vi "UHR-Fleezers Control (host) - 16.2.2v2.vi"() -> ()   [LabVIEW 2014] (continued)
  n239 = call "IMAQ Create"("Image Name"="APD 1 Image", "Image Type"=w48) -> ("New Image"=w71:T2)  [unwired: 3 in, 1 out]
  n240 = call "IMAQ Create"("Image Name"="APD 2 Image", "Image Type"=w48) -> ("New Image"=w70:T2)  [unwired: 3 in, 1 out]
  n241 = call "IMAQ Create"("Image Name"="APD 3 Image", "Image Type"=w48) -> ("New Image"=w47:T2)  [unwired: 3 in, 1 out]
  n242 = call "IMAQ Create"("Image Name"="Det. X Image", "Image Type"=w48) -> ("New Image"=w69:T2)  [unwired: 3 in, 1 out]
  n243 = call "IMAQ Create"("Image Name"="Det. Y Image", "Image Type"=w48) -> ("New Image"=w68:T2)  [unwired: 3 in, 1 out]
  n244 = call-poly "VISA Configure Serial Port"("VISA resource name"=refnum<visa-resource-name> "COM1") -> ("VISA resource name out"=w15:refnum<visa-resource-name>, "error out"=w78:errorcluster)  [unwired: 5 in, 8 out]
  "Stage Control Serial Error" <- w78
  n245 = call-poly "VISA Configure Serial Port"("VISA resource name"=refnum<visa-resource-name> "COM6", "baud rate (9600)"=u32 115200, "stop bits (10: 1 bit)"=w65) -> ("VISA resource name out"=w63:refnum<visa-resource-name>, "error out"=w64:errorcluster)  [unwired: 4 in, 7 out]
  n246 = Bundle("New Image"=w71, "New Image"=w70, "New Image"=w47, "New Image"=w69, "New Image"=w68) -> (w67:T27)  [unwired: 1 in]
  n247 = node-c288() -> (w74:T28)  [unwired: 4 in]
  n248 = node-c288() -> (w87:T28)  [unwired: 4 out]
  n249 = node-c288() -> (w46:T28)  [unwired: 4 out]
  n250 = node-c288(3 ("Processor")) -> (w83:T28)  [unwired: 3 out]
  n251 = node-c288(2 ("Processor")) -> (w85:T28)  [unwired: 3 out]
  n252 = node-c288(i64 1 ("Period"), 1 ("Processor")) -> (w91:T28)  [unwired: 2 out]
  n253 = timed-loop "Run Scripts, including: stage motion" {
    tunnel: w78 -> [w430]
    tunnel: w15 -> [w431]
    tunnel: [w431] -> w77
    tunnel: [w430] -> w76
    timing: w74 -> [_]
    timing-out: [_] -> w73
    tunnel: w63 -> [w429]
    tunnel: w64 -> [w428]
    tunnel: w55 -> [w425]
    tunnel: w54 -> [w424]
    tunnel: w53 -> [w426]
    tunnel: w52 -> [w427]
    tunnel: w42 -> [w423]
    tunnel: w36 -> [w422]
    tunnel: w8 -> [w421]
    tunnel: w5 -> [w420]
    stop <- w432 stop-if-true
    n254 = node-c288() -> ()  [unwired: 1 in, 1 out]
    n255 = event shown="[32] \"Start slow f-ext\": Value Change" {
      selector: _ -> [_ _ _ _ _ _ _ _ _ _ _ _ _ _ _ _ _ _ _ _ _ _ _ _ _ _ _ _ _ _ _ _ _]
      dyn-events: _ -> [_ _ _ _ _ _ _ _ _ _ _ _ _ _ _ _ _ _ _ _ _ _ _ _ _ _ _ _ _ _ _ _ _]
      timeout: _ -> [_ _ _ _ _ _ _ _ _ _ _ _ _ _ _ _ _ _ _ _ _ _ _ _ _ _ _ _ _ _ _ _ _]
      tunnel: ["Set Position" "Move to Position" _ _ _ _ _ _ _ _ "Read Harvard" _ _ _ _ _ _ _ _ "Got ADig bead" "Force FB Data\nScript" _ _ _ "Got DNA bead" "Take Stepping Data" _ "Take Detection Laser\nImage" _ _ _ _ _] -> _
      tunnel: [_ _ _ _ _ _ _ _ _ _ _ _ _ _ _ _ _ _ _ _ _ _ _ _ _ _ _ _ _ w1446 _ _ _] -> w432
      tunnel: w430 -> [w451 w459 w472 w502 _ _ _ _ _ _ _ w646 w680 w706 w738 w832 w861 w993 w1020 _ w1056 _ _ _ _ _ _ _ _ _ _ _ _]
      tunnel: w431 -> [w452 w460 w473 w503 _ _ _ _ _ _ _ w647 w681 w707 w739 w833 w862 w994 w1021 _ w1057 _ _ _ _ _ _ _ _ _ _ _ _]
      tunnel: w429 -> [_ _ _ _ _ _ _ _ _ _ w631 _ _ _ _ _ _ _ _ _ _ _ _ _ _ _ _ _ _ _ _ _ _]
      tunnel: w428 -> [_ _ _ _ _ _ _ _ _ _ w630 _ _ _ _ _ _ _ _ _ _ _ _ _ _ _ _ _ _ _ _ _ _]
      tunnel: w427 -> [_ _ _ _ _ _ _ _ _ _ _ _ _ _ _ _ _ _ _ _ _ _ _ _ _ _ _ _ _ _ _ _ _]
      tunnel: w426 -> [_ _ _ _ _ _ _ _ _ _ _ _ _ _ _ _ _ _ _ _ _ _ _ _ _ _ _ _ _ _ _ _ _]
      tunnel: w425 -> [_ _ _ _ _ _ _ _ _ _ _ _ _ _ _ _ _ _ _ _ _ _ _ _ _ _ _ _ _ _ _ _ _]
      tunnel: w424 -> [_ _ _ _ _ _ _ _ _ _ _ _ _ _ _ _ _ _ _ _ _ _ _ _ _ _ _ _ _ _ _ _ _]
      tunnel: w423 -> [_ _ _ _ w530 w537 w565 w584 _ _ _ _ _ _ _ _ _ _ _ _ _ _ _ _ _ _ _ _ _ w1445 _ _ _]
      tunnel: w422 -> [_ _ _ _ _ _ _ _ _ _ _ _ _ _ _ _ _ _ _ _ _ w1104 w1117 _ _ _ _ _ w1312 _ _ _ _]
      tunnel: w421 -> [_ _ _ _ _ _ _ _ _ _ _ _ _ _ _ _ _ _ _ _ _ _ _ _ _ _ _ _ _ _ w1456 _ _]
      tunnel: w420 -> [_ _ _ _ _ _ _ _ _ _ _ _ _ _ _ _ _ _ _ _ _ _ _ _ _ _ _ _ _ _ w1451 _ _]
      event "Set Position", "Set Position 2", "Set Position 3", "Set Position 4", "Set Position 5", "Set Position 1", "Set Position 6": Value Change {
        n256 = event-data() -> ()  [unwired: 1 in, 5 out]
        n257 = Build Array("Set Position 1", "Set Position 2", "Set Position 3", "Set Position 4", "Set Position 5", "Set Position 6") -> (w450:bool[])
        n258 = Boolean Array To Number(Boolean array=w450) -> (number=w449:u32)
        n259 = Logarithm Base 2(1:w449) -> (0:w441:dbl)
        n260 = call "Read Stage Position.vi"("error in"=w451, "VISA resource name in"=w452) -> ("Current Position"=w456:cluster{dbl, dbl, dbl}, "error out"=w455:errorcluster)  [unwired: 2 out]
        n261 = Decrement(x="Position") -> (x-1=w439:dbl)
        n262 = Greater Or Equal?(x=w441, y=0.0) -> (x >= y?=w442:bool)
        n263 = Cluster To Array(cluster=w456) -> (array=w453:dbl[])
        n264 = local write "Stage Control Serial Error"(w455) -> ()
        n265 = Select(t=w441, s=w442, f=w439) -> (s? t:f=w438:dbl)
        n266 = Increment(x=w438) -> (x+1=w437:dbl)
        n267 = Build Array (concatenate)(w437, w453) -> (w436:dbl[])
        n268 = Replace Array Subset(array="Saved Stage Positions", new element=w436, index (row)=w438) -> (w454:dbl[][])  [unwired: 1 in]
        n269 = local write "Saved Stage Positions"(w454) -> ()
      }
      event "Move to Position": Value Change {
        n270 = event-data() -> ()  [unwired: 1 in, 5 out]
        n271 = flat-sequence {
          tunnel: w460 -> [w464]
          tunnel: w459 -> [w463]
          frame #0 {
            n272 = local read "Saved Stage Positions"() -> (w466:dbl[][])
            n273 = local read "Position"() -> (w465:dbl)
            n274 = local write "Stage Moving"(TRUE ("Stage Moving")) -> ()
            n275 = call "move to saved stage position.vi"("error in"=w463, "Stage VISA resource name in"=w464, "Position"=w465, "Saved Stage Positions"=w466) -> ("error out"=w462:errorcluster)  [unwired: 1 out]
            n276 = local write "Stage Control Serial Error"(w462) -> ()
          }
          frame #1 {
            n277 = call <vilib>:"Beep.vi"() -> ()  [unwired: 3 in, 9 out]
            n278 = local write "Stage Moving"(FALSE ("Stage Moving")) -> ()
          }
        }
      }
      event "Move Cap. 1 (DNA Bottom)": Value Change {
        n279 = event-data() -> ()  [unwired: 1 in, 5 out]
        n280 = local write "Move Cap. 1 (DNA Bottom)"(FALSE ("Move Cap. 1 (DNA Right)")) -> ()
        n281 = flat-sequence {
          tunnel: w472 -> [w475]
          tunnel: w473 -> [w476]
          tunnel: [w476] -> w470
          tunnel: [w475] -> w469
          tunnel: w470 -> [w478]
          tunnel: w469 -> [w477]
          frame #0 {
            n282 = property on="Sample Channel\nFlow" class="Bool (strict)"("Val(Sgnl)"="Cap 1 Samp Flow ON") -> ()  [unwired: 2 in, 2 out]
          }
          frame #1 {
            n283 = local read "Saved Stage Positions"() -> (w488:dbl[][])
            n284 = local write "Stage Moving"(TRUE ("Stage Moving")) -> ()
            n285 = Array Subset(array=w488, index (row)=0 ("index"), length (row)=1 ("length"), index (col)=1 ("index"), length (col)=3 ("length")) -> (w485:dbl[][])
            n286 = Reshape Array(w485, 3 ("dimension size")) -> (w483:dbl[])
            n287 = Array To Cluster(array=w483) -> (cluster=w482:cluster{"[0]":dbl, "[1]":dbl, "[2]":dbl})
            n288 = call "Set Stage Position.vi"("Position"=w482, "error in"=w477, "VISA resource name in"=w478) -> ("error out"=w481:errorcluster)  [unwired: 2 out]
            n289 = local write "Stage Control Serial Error"(w481) -> ()
          }
          frame #2 {
            n290 = local write "Stage Moving"(FALSE ("Stage Moving")) -> ()
            n291 = case shown="True" "Cap 1 Flow ON" {
              frame False {
              }
              frame True {
                n292 = property on="Inject Pump 1" class="Bool (strict)"("Val(Sgnl)"=TRUE ("Value (Signaling)")) -> ()  [unwired: 2 in, 2 out]
              }
            }
            n293 = call <vilib>:"Beep.vi"() -> ()  [unwired: 3 in, 9 out]
          }
          frame #3 {
            n294 = property on="Sample Channel\nFlow" class="Bool (strict)"("Val(Sgnl)"=FALSE ("Value (Signaling)")) -> ()  [unwired: 2 in, 2 out]
            n295 = local read "Cap. 2 BD T1?\n(ADig T1, DNA T2)"() -> (w495:bool)
            n296 = case shown="True" w495 {
              tunnel: "Cap 1 T ON" -> [w497 w498]
              frame False {
                n297 = property on="Trap 1 (ON/OFF)" class="Bool (strict)"("Val(Sgnl)"=w497) -> ()  [unwired: 2 in, 2 out]
              }
              frame True {
                n298 = property on="Trap 2 (ON/OFF)" class="Bool (strict)"("Val(Sgnl)"=w498) -> ()  [unwired: 2 in, 2 out]
              }
            }
            n299 = property on="Got DNA bead" class="Bool"("Key Focus"=TRUE) -> ()  [unwired: 2 in, 2 out]
          }
        }
      }
      event "Move Cap. 2 (ADig Top)": Value Change {
        n300 = event-data() -> ()  [unwired: 1 in, 5 out]
        n301 = local write "Move Cap. 2 (ADig Top)"(FALSE ("Move Cap. 2 (ADig Left)")) -> ()
        n302 = flat-sequence {
          tunnel: w502 -> [w505]
          tunnel: w503 -> [w506]
          tunnel: [w506] -> w500
          tunnel: [w505] -> w499
          tunnel: w500 -> [w509]
          tunnel: w499 -> [w508]
          frame #0 {
            n303 = property on="Sample Channel\nFlow" class="Bool (strict)"("Val(Sgnl)"="Cap 2 Samp Flow ON") -> ()  [unwired: 2 in, 2 out]
          }
          frame #1 {
            w507 = FALSE ("Value (Signaling)")
            n304 = local read "Saved Stage Positions"() -> (w519:dbl[][])
            n305 = local write "Stage Moving"(TRUE ("Stage Moving")) -> ()
            n306 = Array Subset(array=w519, index (row)=1 ("index"), length (row)=1 ("length"), index (col)=1 ("index"), length (col)=3 ("length")) -> (w516:dbl[][])
            n307 = Reshape Array(w516, 3 ("dimension size")) -> (w514:dbl[])
            n308 = property on="Trap 1 (ON/OFF)" class="Bool (strict)"("Val(Sgnl)"=w507) -> ()  [unwired: 2 in, 2 out]
            n309 = property on="Trap 1 (ON/OFF)" class="Bool (strict)"("Val(Sgnl)"=w507) -> ()  [unwired: 2 in, 2 out]
            n310 = Array To Cluster(array=w514) -> (cluster=w513:cluster{"[0]":dbl, "[1]":dbl, "[2]":dbl})
            n311 = call "Set Stage Position.vi"("Position"=w513, "error in"=w508, "VISA resource name in"=w509) -> ("error out"=w512:errorcluster)  [unwired: 2 out]
            n312 = local write "Stage Control Serial Error"(w512) -> ()
          }
          frame #2 {
            n313 = local write "Stage Moving"(FALSE ("Stage Moving")) -> ()
            n314 = call <vilib>:"Beep.vi"() -> ()  [unwired: 3 in, 9 out]
            n315 = case shown="True" "Cap 2 Flow ON" {
              frame False {
              }
              frame True {
                n316 = property on="Inject Pump 3" class="Bool (strict)"("Val(Sgnl)"=TRUE ("Value (Signaling)")) -> ()  [unwired: 2 in, 2 out]
              }
            }
          }
          frame #3 {
            n317 = property on="Sample Channel\nFlow" class="Bool (strict)"("Val(Sgnl)"=FALSE ("Value (Signaling)")) -> ()  [unwired: 2 in, 2 out]
            n318 = case shown="False" "Cap. 2 BD T1?\n(ADig T1, DNA T2)" {
              tunnel: "Cap 2 T ON" -> [w528 w529]
              frame False {
                n319 = property on="Trap 2 (ON/OFF)" class="Bool (strict)"("Val(Sgnl)"=w528) -> ()  [unwired: 2 in, 2 out]
              }
              frame True {
                n320 = property on="Trap 1 (ON/OFF)" class="Bool (strict)"("Val(Sgnl)"=w529) -> ()  [unwired: 2 in, 2 out]
              }
            }
            n321 = property on="Got ADig bead" class="Bool"("Key Focus"=TRUE) -> ()  [unwired: 2 in, 2 out]
          }
        }
      }
      event "Send string\nto Blue Laser": Value Change {
        n322 = event-data() -> ()  [unwired: 1 in, 5 out]
        n323 = flat-sequence {
          tunnel: w530 -> [w531]
          frame #0 {
            n324 = call "serial write macro.vi"("String"="command string", "Delay (ms)"="Delay (ms)", "VISA resource name"=w531) -> ("read buffer"=→"read blue buffer":string, "error out"=→"Blue Error Out":errorcluster)  [unwired: 1 out]
            "command string sent" <- "command string"
          }
          frame #1 {
            n325 = local write "Send string\nto Blue Laser"(FALSE ("Send string")) -> ()
          }
        }
      }
      event "Get Blue Laser State": Value Change {
        n326 = event-data() -> ()  [unwired: 1 in, 5 out]
        n327 = local read "Delay (ms)"() -> (w538:i32)
        n328 = flat-sequence {
          tunnel: w538 -> [w546]
          tunnel: w537 -> [w549]
          tunnel: [w547] -> w542
          tunnel: [w546] -> w541
          tunnel: [w556] -> w540
          tunnel: [w553] -> w539
          tunnel: w542 -> [w554]
          tunnel: w541 -> [w553]
          tunnel: w540 -> [w562]
          tunnel: w539 -> [w560]
          frame #0 {
            w544 = "l?"
            n329 = local write "command string sent"(w544) -> ()
            n330 = call "serial write macro.vi"("String"=w544, "Delay (ms)"=w546, "VISA resource name"=w549) -> ("read buffer"=w545:string, "VISA resource name out"=w547:refnum<visa-resource-name>)  [unwired: 1 out]
            n331 = Decimal String To Number(string=w545) -> (number=w548:i32)  [unwired: 2 in, 1 out]
            n332 = Not Equal To 0?(x=w548) -> (x != 0?=→"Laser On":bool)
            n333 = local write "read blue buffer"(w545) -> ()
          }
          frame #1 {
            w551 = "games?" ("String")
            n334 = local write "command string sent"(w551) -> ()
            n335 = call "serial write macro.vi"("String"=w551, "Delay (ms)"=w553, "VISA resource name"=w554) -> ("read buffer"=w552:string, "VISA resource name out"=w556:refnum<visa-resource-name>)  [unwired: 1 out]
            n336 = Decimal String To Number(string=w552) -> (number=w555:i32)  [unwired: 2 in, 1 out]
            n337 = local write "read blue buffer"(w552) -> ()
            n338 = Not Equal To 0?(x=w555) -> (x != 0?=→"Analog Modulation":bool)
          }
          frame #2 {
            w558 = "gdmes?" ("String")
            n339 = local write "command string sent"(w558) -> ()
            n340 = call "serial write macro.vi"("String"=w558, "Delay (ms)"=w560, "VISA resource name"=w562) -> ("read buffer"=w559:string)  [unwired: 2 out]
            n341 = Decimal String To Number(string=w559) -> (number=w561:i32)  [unwired: 2 in, 1 out]
            n342 = Not Equal To 0?(x=w561) -> (x != 0?=→"Digital Modulation":bool)
            n343 = local write "read blue buffer"(w559) -> ()
          }
          frame #3 {
            n344 = local write "Get Blue Laser State"(FALSE) -> ()
          }
        }
      }
      event "Blue Laser Power (mW)\n(Constant Power Mode)", "Blue Laser Modulation\nPower (mW)": Value Change {
        n345 = event-data() -> ()  [unwired: 1 in, 5 out]
        n346 = flat-sequence {
          tunnel: w565 -> [w571]
          tunnel: [w569] -> w564
          tunnel: w564 -> [w578]
          frame #0 {
            n347 = local read "Delay (ms)"() -> (w570:i32)
            n348 = Concatenate Strings("slmp " ("string"), "Blue Laser Modulation\nPower (mW)") -> (w566:string)
            n349 = call "serial write macro.vi"("String"=w566, "Delay (ms)"=w570, "VISA resource name"=w571) -> ("read buffer"=w567:string, "error out"=w568:errorcluster, "VISA resource name out"=w569:refnum<visa-resource-name>)
            n350 = local write "command string sent"(w566) -> ()
            n351 = local write "read blue buffer"(w567) -> ()
            n352 = local write "Blue Error Out"(w568) -> ()
          }
          frame #1 {
            n353 = local read "Delay (ms)"() -> (w577:i32)
            n354 = Concatenate Strings("p " ("string"), "Blue Laser Power (mW)\n(Constant Power Mode)") -> (w574:string)
            n355 = call "serial write macro.vi"("String"=w574, "Delay (ms)"=w577, "VISA resource name"=w578) -> ("read buffer"=w575:string, "error out"=w576:errorcluster)  [unwired: 1 out]
            n356 = local write "command string sent"(w574) -> ()
            n357 = local write "read blue buffer"(w575) -> ()
            n358 = local write "Blue Error Out"(w576) -> ()
          }
        }
      }
      event "Laser interlacing mode", "Blue Laser Modulation Mode", "Blue Laser ON": Value Change {
        n359 = event-data() -> ()  [unwired: 1 in, 5 out]
        n360 = flat-sequence {
          tunnel: w584 -> [w589]
          tunnel: [w588] -> w581
          tunnel: [w594] -> w583
          tunnel: w581 -> [w597]
          tunnel: w583 -> [w609]
          tunnel: [w603] -> w582
          tunnel: w582 -> [w616]
          frame #0 {
            n361 = local read "Blue Laser ON"() -> (w586:bool)
            n362 = local read "Delay (ms)"() -> (w587:i32)
            n363 = case shown="False" w586 {
              tunnel: ["l0" "l1"] -> w585
              frame False {
              }
              frame True {
              }
            }
            n364 = call "serial write macro.vi"("String"=w585, "Delay (ms)"=w587, "VISA resource name"=w589) -> ("error out"=w590:errorcluster, "VISA resource name out"=w588:refnum<visa-resource-name>)  [unwired: 1 out]
            n365 = local write "Blue Error Out"(w590) -> ()
          }
          frame #1 {
            n366 = local read "Laser interlacing mode"() -> (w599:enum32{"Laser ON", "Laser OFF", "Interlace"})
            n367 = case shown="\"Laser ON\"" w599 {
              tunnel: ["cp" "em" "l0"] -> w593
              frame "Laser ON" {
              }
              frame "Interlace" {
              }
              frame "Laser OFF", Default {
              }
            }
            n368 = local read "Delay (ms)"() -> (w598:i32)
            n369 = call "serial write macro.vi"("String"=w593, "Delay (ms)"=w598, "VISA resource name"=w597) -> ("read buffer"=w595:string, "error out"=w596:errorcluster, "VISA resource name out"=w594:refnum<visa-resource-name>)
            n370 = local write "command string sent"(w593) -> ()
            n371 = local write "read blue buffer"(w595) -> ()
            n372 = local write "Blue Error Out"(w596) -> ()
          }
          frame #2 {
            n373 = case shown="\"Analog Modulation\"" "Blue Laser Modulation Mode" {
              tunnel: ["sdmes 0" "sdmes 1" "sdmes 1"] -> w604
              frame "Analog Modulation" {
              }
              frame "Digital + Analog Modulation" {
              }
              frame "Digital Modulation", Default {
              }
            }
            n374 = local read "Delay (ms)"() -> (w607:i32)
            n375 = call "serial write macro.vi"("String"=w604, "Delay (ms)"=w607, "VISA resource name"=w609) -> ("read buffer"=w605:string, "error out"=w606:errorcluster, "VISA resource name out"=w603:refnum<visa-resource-name>)
            n376 = local write "command string sent"(w604) -> ()
            n377 = local write "read blue buffer"(w605) -> ()
            n378 = local write "Blue Error Out"(w606) -> ()
          }
          frame #3 {
            n379 = local read "Blue Laser Modulation Mode"() -> (w618:string)
            n380 = case shown="\"Digital Modulation\", Default" w618 {
              tunnel: ["sames 1" "sames 1" "sames 0"] -> w614
              frame "Analog Modulation" {
              }
              frame "Digital + Analog Modulation" {
              }
              frame "Digital Modulation", Default {
              }
            }
            n381 = local read "Delay (ms)"() -> (w617:i32)
            n382 = local write "command string sent"(w614) -> ()
            n383 = call "serial write macro.vi"("String"=w614, "Delay (ms)"=w617, "VISA resource name"=w616) -> ("read buffer"=w615:string, "error out"=w613:errorcluster)  [unwired: 1 out]
            n384 = local write "read blue buffer"(w615) -> ()
            n385 = local write "Blue Error Out"(w613) -> ()
          }
        }
      }
      event "All excitation lasers OFF": Value Change {
        n386 = event-data() -> ()  [unwired: 1 in, 5 out]
        n387 = flat-sequence {
          frame #0 {
            w623 = FALSE ("Red Laser ON")
            n388 = local write "All excitation lasers OFF"(FALSE ("All excitation lasers OFF")) -> ()
            n389 = local write "Blue Laser ON"(w623) -> ()
            n390 = local write "Red Laser ON"(w623) -> ()
          }
          frame #1 {
            n391 = property on="Green Laser ON" class="Bool (strict)"("Val(Sgnl)"=FALSE ("Value (Signaling)")) -> ()  [unwired: 2 in, 2 out]
          }
        }
      }
      event "Start ALEX": Value Change {
        n392 = event-data() -> ()  [unwired: 1 in, 5 out]
        n393 = flat-sequence {
          frame #0 {
            n394 = property on="ALEX ON" class="Bool (strict)"("Val(Sgnl)"=FALSE ("Value (Signaling)")) -> ()  [unwired: 2 in, 2 out]
          }
          frame #1 {
            w626 = TRUE ("Value (Signaling)")
            n395 = local write "Red Laser ON"(w626) -> ()
            n396 = local write "Start ALEX"(FALSE ("Start ALEX")) -> ()
            n397 = property on="ALEX ON" class="Bool (strict)"("Val(Sgnl)"=w626) -> ()  [unwired: 2 in, 2 out]
          }
          frame #2 {
            n398 = property on="Green Laser ON" class="Bool (strict)"("Val(Sgnl)"=TRUE ("Value (Signaling)")) -> ()  [unwired: 2 in, 2 out]
          }
        }
      }
      event "Read Harvard": Value Change {
        n399 = event-data() -> ()  [unwired: 1 in, 5 out]
        n400 = Concatenate Strings("write buffer", "\r") -> (w633:string)
        n401 = VISA Write(VISA resource name=w631, write buffer=w633, error in (no error)=w630) -> (VISA resource name out=w642:refnum<visa-resource-name>, error out=w641:errorcluster)  [unwired: 1 out]
        n402 = stacked-sequence {
          tunnel: [w645] -> w640
          tunnel: w642 -> [w645]
          tunnel: w641 -> [w644]
          tunnel: [w644] -> w635
          frame #0 {
            n403 = Wait (ms)(milliseconds to wait=50) -> ()  [unwired: 1 out]
          }
        }
        n404 = property class="Instr"(reference=w640, error in=w635) -> (reference out=w639:refnum<visa-resource-name>, error out=w637:errorcluster, "Serial Settings:Number of Bytes at Serial Port"=w638:u32)
        "Serial Settings:Number of Bytes at Serial Port" <- w638
        n405 = VISA Read(VISA resource name=w639, byte count=w638, error in (no error)=w637) -> (read buffer=w636:string)  [unwired: 3 out]
        "read buffer" <- w636
        n406 = Fract/Exp String To Number(string=w636) -> ()  [unwired: 5 out]
      }
      event "+z", "-z": Value Change {
        n407 = event-data() -> ()  [unwired: 1 in, 5 out]
        n408 = flat-sequence {
          tunnel: w646 -> [w668]
          tunnel: w647 -> [w648]
          frame #0 {
            n409 = call "Read Stage Position.vi"("error in"=w668, "VISA resource name in"=w648) -> ("Current Position"=w653:cluster{dbl, dbl, dbl}, "error out"=w666:errorcluster, "VISA resource name out"=w667:refnum<visa-resource-name>)  [unwired: 1 out]
            n410 = local read "Saved Stage Positions"() -> (w677:dbl[][])
            n411 = Divide(x="z nudge increment (um)", y=1000.0) -> (x/y=w665:dbl)
            n412 = Boolean To (0,1)(Boolean="+z") -> (0, 1=w657:i16)
            n413 = Boolean To (0,1)(Boolean="-z") -> (0, 1=w658:i16)
            n414 = Array Subset(array=w677, index (row)=1 ("index"), length (row)=1 ("length"), index (col)=1 ("index"), length (col)=3 ("length")) -> (w674:dbl[][])
            n415 = Multiply(x=w657, y=w665) -> (x*y=w661:dbl)
            n416 = Multiply(x=w658, y=w665) -> (x*y=w659:dbl)
            n417 = Unbundle(w653) -> (w651:dbl, w650:dbl, w654:dbl)
            n418 = Negate(x=w659) -> (-x=w660:dbl)
            n419 = Reshape Array(w674, 3 ("dimension size")) -> (w672:dbl[])
            n420 = Add(x=w661, y=w660) -> (x+y=w662:dbl)
            n421 = Array To Cluster(array=w672) -> ()  [unwired: 1 out]
            n422 = Add(x=w662, y=w654) -> (x+y=w652:dbl)
            n423 = Bundle(cluster=w653, w651, w650, w652) -> (w649:cluster{dbl, dbl, dbl})
            n424 = call "Set Stage Position.vi"("Position"=w649, "error in"=w666, "VISA resource name in"=w667) -> ("error out"=w671:errorcluster)  [unwired: 2 out]
            n425 = local write "Stage Moving"(TRUE ("Stage Moving")) -> ()
            n426 = local write "Stage Control Serial Error"(w671) -> ()
          }
          frame #1 {
            n427 = local write "Stage Moving"(FALSE ("Stage Moving")) -> ()
          }
        }
      }
      event "-y", "+y": Value Change {
        n428 = event-data() -> ()  [unwired: 1 in, 5 out]
        n429 = flat-sequence {
          tunnel: w680 -> [w704]
          tunnel: w681 -> [w687]
          frame #0 {
            n430 = call "Read Stage Position.vi"("error in"=w704, "VISA resource name in"=w687) -> ("Current Position"=w690:cluster{dbl, dbl, dbl}, "error out"=w702:errorcluster, "VISA resource name out"=w703:refnum<visa-resource-name>)  [unwired: 1 out]
            n431 = Divide(x="y nudge increment (um", y=1000.0) -> (x/y=w701:dbl)
            n432 = Boolean To (0,1)(Boolean="+y") -> (0, 1=w693:i16)
            n433 = Boolean To (0,1)(Boolean="-y") -> (0, 1=w694:i16)
            n434 = Multiply(x=w693, y=w701) -> (x*y=w697:dbl)
            n435 = Multiply(x=w694, y=w701) -> (x*y=w695:dbl)
            n436 = Unbundle(w690) -> (w689:dbl, w684:dbl, w686:dbl)
            n437 = Negate(x=w695) -> (-x=w696:dbl)
            n438 = Add(x=w697, y=w696) -> (x+y=w698:dbl)
            n439 = Add(x=w698, y=w684) -> (x+y=w685:dbl)
            n440 = Bundle(cluster=w690, w689, w685, w686) -> (w688:cluster{dbl, dbl, dbl})
            n441 = call "Set Stage Position.vi"("Position"=w688, "error in"=w702, "VISA resource name in"=w703) -> ("error out"=w683:errorcluster)  [unwired: 2 out]
            n442 = local write "Stage Control Serial Error"(w683) -> ()
            n443 = local write "Stage Moving"(TRUE ("Stage Moving")) -> ()
          }
          frame #1 {
            n444 = local write "Stage Moving"(FALSE ("Stage Moving")) -> ()
          }
        }
      }
      event "-x", "+x": Value Change {
        n445 = event-data() -> ()  [unwired: 1 in, 5 out]
        n446 = flat-sequence {
          tunnel: w706 -> [w730]
          tunnel: w707 -> [w714]
          frame #0 {
            n447 = call "Read Stage Position.vi"("error in"=w730, "VISA resource name in"=w714) -> ("Current Position"=w716:cluster{dbl, dbl, dbl}, "error out"=w728:errorcluster, "VISA resource name out"=w729:refnum<visa-resource-name>)  [unwired: 1 out]
            n448 = Divide(x="x nudge increment (um)", y=1000.0) -> (x/y=w727:dbl)
            n449 = Boolean To (0,1)(Boolean="+x") -> (0, 1=w719:i16)
            n450 = Boolean To (0,1)(Boolean="-x") -> (0, 1=w720:i16)
            n451 = Multiply(x=w719, y=w727) -> (x*y=w723:dbl)
            n452 = Multiply(x=w720, y=w727) -> (x*y=w721:dbl)
            n453 = Unbundle(w716) -> (w708:dbl, w710:dbl, w713:dbl)
            n454 = Negate(x=w721) -> (-x=w722:dbl)
            n455 = Add(x=w723, y=w722) -> (x+y=w724:dbl)
            n456 = Add(x=w724, y=w708) -> (x+y=w709:dbl)
            n457 = Bundle(cluster=w716, w709, w710, w713) -> (w715:cluster{dbl, dbl, dbl})
            n458 = call "Set Stage Position.vi"("Position"=w715, "error in"=w728, "VISA resource name in"=w729) -> ("error out"=w711:errorcluster)  [unwired: 2 out]
            n459 = local write "Stage Control Serial Error"(w711) -> ()
            n460 = local write "Stage Moving"(TRUE ("Stage Moving")) -> ()
          }
          frame #1 {
            n461 = local write "Stage Moving"(FALSE ("Stage Moving")) -> ()
          }
        }
      }
      event "Cal/Data Acq. Spot": Value Change {
        n462 = event-data() -> ()  [unwired: 1 in, 5 out]
        n463 = flat-sequence {
          tunnel: w738 -> [w742]
          tunnel: w739 -> [w743]
          tunnel: [w743] -> w735
          tunnel: [w742] -> w734
          tunnel: w735 -> [w748]
          tunnel: w734 -> [w747]
          tunnel: ["Cal @ (MHz)"] -> w732
          tunnel: [w752] -> w736
          tunnel: w732 -> [w752]
          tunnel: w736 -> [w764]
          tunnel: ["W/ Offset 1"] -> w733
          tunnel: w736 -> [w785]
          tunnel: w733 -> [w783]
          frame #0 {
            n464 = property on="Sample Channel\nFlow" class="Bool (strict)"("Val(Sgnl)"="Daq spot flow on") -> ()  [unwired: 2 in, 2 out]
            n465 = Wait (ms)(milliseconds to wait=u32 250) -> ()  [unwired: 1 out]
          }
          frame #1 {
            n466 = local read "Saved Stage Positions"() -> (w745:dbl[][])
            n467 = property on="Trap Delta (MHz)" class="DigNum (strict)"("Val(Sgnl)"="Cal @ (MHz)") -> ()  [unwired: 2 in, 2 out]
            n468 = local write "Stage Moving"(TRUE ("Stage Moving")) -> ()
            n469 = call "move to saved stage position.vi"("error in"=w747, "Stage VISA resource name in"=w748, "Position"="Cal Stage Position", "Saved Stage Positions"=w745) -> ("error out"=w746:errorcluster)  [unwired: 1 out]
            n470 = local write "Stage Control Serial Error"(w746) -> ()
          }
          frame #2 {
            n471 = local write "Stage Moving"(FALSE ("Stage Moving")) -> ()
            n472 = property on="Sample Channel\nFlow" class="Bool (strict)"("Val(Sgnl)"="Flow ON during cal?") -> ()  [unwired: 2 in, 2 out]
            n473 = call <vilib>:"Beep.vi"() -> ()  [unwired: 3 in, 9 out]
          }
          frame #3 {
            n474 = Wait (ms)(milliseconds to wait=u32 1000) -> ()  [unwired: 1 out]
          }
          frame #4 {
            n475 = case shown="True" "Active cal after cal?" {
              frame False {
              }
              frame True {
                n476 = local write "Active Cal"(TRUE ("Active Cal")) -> ()
                n477 = Wait (ms)(milliseconds to wait=u32 8000) -> ()  [unwired: 1 out]
              }
            }
          }
          frame #5 {
            n478 = property on="Save Calibration" class="Bool (strict)"("Val(Sgnl)"=TRUE ("Value (Signaling)")) -> ()  [unwired: 2 in, 2 out]
          }
          frame #6 {
            n479 = Wait (ms)(milliseconds to wait=u32 2000) -> ()  [unwired: 1 out]
          }
          frame #7 {
            # "Check to see if \nsaving done"
            n480 = while {
              stop <- w760 stop-if-true
              n481 = local read "Saving..."() -> (w761:bool)
              n482 = Wait (ms)(milliseconds to wait=u32 100) -> ()  [unwired: 1 out]
              n483 = Not(x=w761) -> (.not. x?=w760:bool)
            }
          }
          frame #8 {
            n484 = case shown="True" "W/ Offset 1" {
              tunnel: w764 -> [_ w765]
              frame False {
              }
              frame True {
                n485 = stacked-sequence {
                  tunnel: w765 -> [_ _ _ _ _ _ _ w782]
                  frame #0 {
                    n486 = property on="Trap Delta (MHz)" class="DigNum (strict)"("Val(Sgnl)"="Offset 1 Start (MHz)") -> ()  [unwired: 2 in, 2 out]
                    n487 = Replace Array Subset(array=u32[] [0] ("Index Values"), new element="Offset 1 Set", index=0) -> (w766:u32[])
                    n488 = property on="Saved AOD Raster Scan Parameter Sets" class="Arr (strict)"("Index Values"=w766) -> ()  [unwired: 2 in, 2 out]
                  }
                  frame #1 {
                    n489 = Wait (ms)(milliseconds to wait=u32 200) -> ()  [unwired: 1 out]
                  }
                  frame #2 {
                    n490 = property on="Load parameters" class="Bool (strict)"("Val(Sgnl)"=TRUE ("Value (Signaling)")) -> ()  [unwired: 2 in, 2 out]
                  }
                  frame #3 {
                    n491 = Wait (ms)(milliseconds to wait=u32 200) -> ()  [unwired: 1 out]
                  }
                  frame #4 {
                    n492 = property on="Trap Raster Scan" class="Bool (strict)"("Val(Sgnl)"=TRUE ("Value (Signaling)")) -> ()  [unwired: 2 in, 2 out]
                  }
                  frame #5 {
                    n493 = Wait (ms)(milliseconds to wait=u32 2000) -> ()  [unwired: 1 out]
                  }
                  frame #6 {
                    n494 = while {
                      stop <- w779 stop-if-true
                      n495 = local read "Raster Scanning..."() -> (w781:bool)
                      n496 = local read "Saving..."() -> (w777:bool)
                      n497 = Wait (ms)(milliseconds to wait=u32 100) -> ()  [unwired: 1 out]
                      n498 = Not(x=w777) -> (.not. x?=w776:bool)
                      n499 = Not(x=w781) -> (.not. x?=w778:bool)
                      n500 = And(x=w778, y=w776) -> (x .and. y?=w779:bool)
                    }
                  }
                  frame #7 {
                    n501 = property on="Trap Delta (MHz)" class="DigNum (strict)"("Val(Sgnl)"=w782) -> ()  [unwired: 2 in, 2 out]
                  }
                }
              }
            }
          }
          frame #9 {
            n502 = local read "Save ave N"() -> (w784:dbl)
            n503 = case shown="False" "W/ Offset 2" {
              tunnel: w785 -> [_ w792]
              tunnel: w784 -> [_ w791]
              tunnel: w783 -> [w787 _]
              frame False {
                n504 = case shown="False" w787 {
                  frame False {
                    n505 = Multiply(x="Cal read wait (s)", y=u32 1000 ("milliseconds to wait")) -> (x*y=w789:u32)
                    n506 = Wait (ms)(milliseconds to wait=w789) -> ()  [unwired: 1 out]
                  }
                  frame True {
                  }
                }
              }
              frame True {
                n507 = stacked-sequence {
                  tunnel: w792 -> [_ _ _ _ _ _ _ _ _ w813 _ _]
                  tunnel: w791 -> [_ _ _ _ _ _ _ _ _ w811 _ _]
                  frame #0 {
                    n508 = property on="Save ave N" class="DigNum (strict)"("Val(Sgnl)"=1.0 ("Value (Signaling)")) -> ()  [unwired: 2 in, 2 out]
                  }
                  frame #1 {
                    n509 = Wait (ms)(milliseconds to wait=u32 500) -> ()  [unwired: 1 out]
                  }
                  frame #2 {
                    n510 = property on="Trap Delta (MHz)" class="DigNum (strict)"("Val(Sgnl)"="Offset 2 Start (MHz)") -> ()  [unwired: 2 in, 2 out]
                    n511 = Replace Array Subset(array=u32[] [0] ("Index Values"), new element="Offset 2 Set", index=0) -> (w797:u32[])
                    n512 = property on="Saved AOD Raster Scan Parameter Sets" class="Arr (strict)"("Index Values"=w797) -> ()  [unwired: 2 in, 2 out]
                  }
                  frame #3 {
                    n513 = Wait (ms)(milliseconds to wait=u32 500) -> ()  [unwired: 1 out]
                  }
                  frame #4 {
                    n514 = property on="Load parameters" class="Bool (strict)"("Val(Sgnl)"=TRUE ("Value (Signaling)")) -> ()  [unwired: 2 in, 2 out]
                  }
                  frame #5 {
                    n515 = Wait (ms)(milliseconds to wait=u32 500) -> ()  [unwired: 1 out]
                  }
                  frame #6 {
                    n516 = property on="Trap Raster Scan" class="Bool (strict)"("Val(Sgnl)"=TRUE ("Value (Signaling)")) -> ()  [unwired: 2 in, 2 out]
                  }
                  frame #7 {
                    n517 = Wait (ms)(milliseconds to wait=u32 2000) -> ()  [unwired: 1 out]
                  }
                  frame #8 {
                    n518 = while {
                      stop <- w806 stop-if-true
                      n519 = local read "Raster Scanning..."() -> (w809:bool)
                      n520 = local read "Saving..."() -> (w807:bool)
                      n521 = Wait (ms)(milliseconds to wait=u32 100) -> ()  [unwired: 1 out]
                      n522 = Not(x=w807) -> (.not. x?=w805:bool)
                      n523 = Not(x=w809) -> (.not. x?=w808:bool)
                      n524 = And(x=w808, y=w805) -> (x .and. y?=w806:bool)
                    }
                  }
                  frame #9 {
                    n525 = property on="Trap Delta (MHz)" class="DigNum (strict)"("Val(Sgnl)"=w813) -> ()  [unwired: 2 in, 2 out]
                    n526 = property on="Saved AOD Raster Scan Parameter Sets" class="Arr (strict)"("Index Values"=u32[] [0]) -> ()  [unwired: 2 in, 2 out]
                    n527 = property on="Save ave N" class="DigNum (strict)"("Val(Sgnl)"=w811) -> ()  [unwired: 2 in, 2 out]
                  }
                  frame #10 {
                    n528 = Wait (ms)(milliseconds to wait=u32 500) -> ()  [unwired: 1 out]
                  }
                  frame #11 {
                    n529 = property on="Load parameters" class="Bool (strict)"("Val(Sgnl)"=TRUE ("Value (Signaling)")) -> ()  [unwired: 2 in, 2 out]
                  }
                }
              }
            }
          }
          frame #10 {
            n530 = property on="Read Cal" class="Bool (strict)"("Val(Sgnl)"=TRUE ("Value (Signaling)")) -> ()  [unwired: 2 in, 2 out]
          }
          frame #11 {
            n531 = Wait (ms)(milliseconds to wait=u32 1000) -> ()  [unwired: 1 out]
          }
          frame #12 {
            # "option to switch fluorescent laser excitation setting\n(to randomize for flurophore bleaching lifetime measurements)"
            n532 = property on="Fish for Tether" class="Bool (strict)"("Val(Sgnl)"="Fish after cal?") -> ()  [unwired: 2 in, 2 out]
            n533 = case shown="True" "Cycle fl ex sp" {
              frame False {
              }
              frame True {
                w826 = 0
                n534 = Array Size(array="Setpoint values (mV)") -> (size(s)=w828:i32)
                n535 = feedback #1(w826) -> (w821:i32)
                n536 = Increment(x=w821) -> (x+1=w820:i32)
                n537 = Equal?(x=w828, y=w820) -> (x = y?=w827:bool)
                n538 = Select(t=w826, s=w827, f=w820) -> (s? t:f=w825:i32)
                n539 = feedback-in #1(w825) -> ()
                n540 = Index Array(array="Setpoint values (mV)", index=w821) -> (element=w822:dbl)
                n541 = property on="Green FB Setpoint (mV)" class="DigNum (strict)"("Val(Sgnl)"=w822) -> ()  [unwired: 2 in, 2 out]
                n542 = Number To Decimal String(number=w822) -> (decimal integer string=w823:string)  [unwired: 1 in]
                n543 = local write "Comment (data description)"(w823) -> ()
              }
            }
          }
        }
        n544 = local write "Cal/Data Acq. Spot"(FALSE ("Cal/Data Acq. Spot")) -> ()
      }
      event "Dump Beads": Value Change {
        n545 = event-data() -> ()  [unwired: 1 in, 5 out]
        n546 = flat-sequence {
          tunnel: ["Dump spot flow on?"] -> w829
          tunnel: [w840] -> w830
          tunnel: w829 -> [w840]
          tunnel: w833 -> [w845]
          tunnel: w832 -> [w844]
          tunnel: [w842] -> w831
          tunnel: w830 -> [w842]
          tunnel: w831 -> [w855]
          frame #0 {
            w834 = FALSE ("Value (Signaling)")
            n547 = local read "Saving..."() -> (w836:bool)
            n548 = local write "Dump Beads"(FALSE ("Dump Beads")) -> ()
            n549 = property on="Inject Pump 3" class="Bool (strict)"("Val(Sgnl)"=w834) -> ()  [unwired: 2 in, 2 out]
            n550 = property on="Inject Pump 1" class="Bool (strict)"("Val(Sgnl)"=w834) -> ()  [unwired: 2 in, 2 out]
            n551 = local write "Stop Saving"(w836) -> ()
          }
          frame #1 {
            w837 = FALSE ("Fl. Triggered...")
            n552 = case shown="True" "Dump spot flow on?" {
              frame False {
              }
              frame True {
                n553 = property on="Sample Channel\nFlow" class="Bool (strict)"("Val(Sgnl)"=TRUE ("Stage Moving")) -> ()  [unwired: 2 in, 2 out]
              }
            }
            n554 = local write "Fl. Triggered..."(w837) -> ()
            n555 = local write "Tether"(w837) -> ()
            n556 = property on="Green Laser ON" class="Bool (strict)"("Val(Sgnl)"=w837) -> ()  [unwired: 2 in, 2 out]
            n557 = property on="Trap Pos. FB ON" class="Bool (strict)"("Val(Sgnl)"=w837) -> ()  [unwired: 2 in, 2 out]
            n558 = property on="Trap Trig. Fl." class="Bool (strict)"("Val(Sgnl)"=w837) -> ()  [unwired: 2 in, 2 out]
            n559 = property on="Fl. Triggered..." class="Bool (strict)"("Val(Sgnl)"=w837) -> ()  [unwired: 2 in, 2 out]
            n560 = property on="Dip for Protein" class="Bool (strict)"("Val(Sgnl)"=w837) -> ()  [unwired: 2 in, 2 out]
            n561 = property on="Pause dwell" class="Bool (strict)"("Val(Sgnl)"=w837) -> ()  [unwired: 2 in, 2 out]
          }
          frame #2 {
            n562 = property on="Trap Pos. FB Offset Factor" class="DigNum (strict)"("Val(Sgnl)"=i64 0 ("Value (Signaling)")) -> ()  [unwired: 2 in, 2 out]
          }
          frame #3 {
            n563 = local read "Saved Stage Positions"() -> (w846:dbl[][])
            n564 = local write "Stage Moving"(TRUE ("Stage Moving")) -> ()
            n565 = Array Subset(array=w846, index (row)=3 ("index"), length (row)=1 ("length"), index (col)=1 ("index"), length (col)=3 ("length")) -> (w851:dbl[][])
            n566 = Reshape Array(w851, 3 ("dimension size")) -> (w849:dbl[])
            n567 = Array To Cluster(array=w849) -> (cluster=w848:cluster{"[0]":dbl, "[1]":dbl, "[2]":dbl})
            n568 = call "Set Stage Position.vi"("Position"=w848, "error in"=w844, "VISA resource name in"=w845) -> ()  [unwired: 3 out]
          }
          frame #4 {
            w856 = FALSE ("Value (Signaling)")
            n569 = case shown="True" w855 {
              frame False {
              }
              frame True {
                n570 = property on="Sample Channel\nFlow" class="Bool (strict)"("Val(Sgnl)"=FALSE ("Stage Moving")) -> ()  [unwired: 2 in, 2 out]
              }
            }
            n571 = property on="Trap 1 (ON/OFF)" class="Bool (strict)"("Val(Sgnl)"=w856) -> ()  [unwired: 2 in, 2 out]
            n572 = property on="Trap 2 (ON/OFF)" class="Bool (strict)"("Val(Sgnl)"=w856) -> ()  [unwired: 2 in, 2 out]
            n573 = call <vilib>:"Beep.vi"() -> ()  [unwired: 3 in, 9 out]
          }
          frame #5 {
            n574 = property on="Move Cap. 2 (ADig Top)" class="Bool (strict)"("Val(Sgnl)"=TRUE ("Value (Signaling)")) -> ()  [unwired: 2 in, 2 out]
            n575 = property on="Tab Control" class="TabCtl (strict)"("Val(Sgnl)"=T31."Status" ("Value (Signaling)")) -> ()  [unwired: 2 in, 2 out]
          }
        }
      }
      event "Dip for Protein": Value Change {
        n576 = event-data() -> ()  [unwired: 1 in, 5 out]
        n577 = case shown="True" "Dip for Protein" {
          tunnel: w862 -> [_ w864]
          tunnel: w861 -> [_ w863]
          frame False {
          }
          frame True {
            n578 = while {
              tunnel: w864 -> [w875]
              tunnel: w863 -> [w874]
              i -> [w869]
              stop <- w871 stop-if-true
              n579 = Increment(x=w869) -> (x+1=→"Dip #":i32)
              n580 = flat-sequence {
                tunnel: w874 -> [w886]
                tunnel: w875 -> [w887]
                tunnel: [w887] -> w879
                tunnel: [w886] -> w878
                tunnel: [w880] -> w865
                tunnel: [w892] -> w873
                tunnel: [w893] -> w872
                tunnel: w879 -> [w894]
                tunnel: w878 -> [w895]
                tunnel: [w890] -> w866
                tunnel: w865 -> [w890]
                tunnel: [w903] -> w877
                tunnel: w873 -> [w903]
                tunnel: [w902] -> w876
                tunnel: w872 -> [w902]
                tunnel: [w899] -> w870
                tunnel: [w898] -> w867
                tunnel: w866 -> [w898]
                tunnel: w876 -> [w923]
                tunnel: w877 -> [w924]
                tunnel: w870 -> [w925]
                tunnel: w867 -> [w922]
                tunnel: [w981] -> w871
                frame #0 {
                  n581 = local read "Trap Pos. FB ON"() -> (w880:bool)
                  n582 = Compound Arithmetic op=AND("Flow ON\nduring dip?", "FB OFF when \nflow ON", w880) -> (w881:bool)
                  n583 = case shown="True" "Move trap \nbefore dip move?" {
                    frame False {
                    }
                    frame True {
                      n584 = property on="Trap Delta (MHz)" class="DigNum (strict)"("Val(Sgnl)"="Dipping Delta (MHz)") -> ()  [unwired: 2 in, 2 out]
                    }
                  }
                  n585 = property on="Green Laser ON" class="Bool (strict)"("Val(Sgnl)"="Green ON\nbefore dip?") -> ()  [unwired: 2 in, 2 out]
                  n586 = property on="Sample Channel\nFlow" class="Bool (strict)"("Val(Sgnl)"="Flow ON\nduring dip?") -> ()  [unwired: 2 in, 2 out]
                  n587 = case shown="True" w881 {
                    frame False {
                    }
                    frame True {
                      n588 = property on="Trap Pos. FB ON" class="Bool (strict)"("Val(Sgnl)"=FALSE ("Value (Signaling)")) -> ()  [unwired: 2 in, 2 out]
                    }
                  }
                }
                frame #1 {
                  n589 = local read "Saved Stage Positions"() -> (w897:dbl[][])
                  n590 = local write "Cancel dwell"(FALSE ("Cancel dwell")) -> ()
                  n591 = call "move to saved stage position.vi"("error in"=w895, "Stage VISA resource name in"=w894, "Position"="Dip Stage \nPosition", "Saved Stage Positions"=w897) -> ("VISA resource name out"=w892:refnum<visa-resource-name>, "error out"=w893:errorcluster)
                }
                frame #2 {
                  n592 = node-c288() -> (w901:T28)  [unwired: 4 in]
                  n593 = timed-loop {
                    timing: w901 -> [_]
                    timing-out: [_] -> w900
                    tunnel: [w907] -> w899
                    i -> [w904]
                    stop <- w908 stop-if-true
                    n594 = node-c288() -> ()  [unwired: 1 in, 1 out]
                    n595 = Greater Or Equal?(x=w904, y="Dip Duration (s)") -> (x >= y?=w916:bool)
                    n596 = local read "Dip for Protein"() -> (w909:bool)
                    n597 = local read "Dump Beads"() -> (w906:bool)
                    n598 = local read "Cancel dwell"() -> (w915:bool)
                    n599 = local read "Pause dwell"() -> (w912:bool)
                    n600 = Not(x=w909) -> (.not. x?=w914:bool)
                    n601 = Compound Arithmetic op=OR(w915, w916, w914) -> (w913:bool)
                    n602 = Select(t=FALSE, s=w912, f=w913) -> (s? t:f=w910:bool)
                    n603 = Not(x=w906) -> (.not. x?=w905:bool)
                    n604 = node-c288() -> ()  [unwired: 1 in, 1 out]
                    n605 = And(x=w909, y=w905) -> (x .and. y?=w907:bool)
                    n606 = Or(x=w910, y=w906) -> (x .or. y?=w908:bool)
                    "Dip Time (s)" <- w904
                  }
                  n607 = node-c288(w900) -> ()  [unwired: 1 out]
                }
                frame #3 {
                  n608 = case shown="True" w925 {
                    tunnel: w924 -> [_ w930]
                    tunnel: w923 -> [_ w929]
                    tunnel: w922 -> [_ w926]
                    frame False {
                    }
                    frame True {
                      n609 = flat-sequence {
                        tunnel: w929 -> [w934]
                        tunnel: w930 -> [w935]
                        tunnel: [w935] -> w928
                        tunnel: [w934] -> w927
                        tunnel: w926 -> [w931]
                        tunnel: w928 -> [w945]
                        tunnel: w927 -> [w944]
                        tunnel: w926 -> [w953]
                        frame #0 {
                          n610 = local read "Sample Channel\nFlow"() -> (w933:bool)
                          n611 = case shown="True" w933 {
                            tunnel: "Flow ON \nduring return\nfrom dip?" -> [w936 w939]
                            tunnel: w931 -> [_ w938]
                            frame False {
                              n612 = case shown="True" w936 {
                                frame False {
                                }
                                frame True {
                                n613 = property on="Sample Channel\nFlow" class="Bool (strict)"("Val(Sgnl)"=TRUE ("Value (Signaling)")) -> ()  [unwired: 2 in, 2 out]
                                }
                              }
                            }
                            frame True {
                              n614 = case shown="False" w939 {
                                tunnel: w938 -> [w940 _]
                                frame False {
                                n615 = property on="Trap Pos. FB ON" class="Bool (strict)"("Val(Sgnl)"=w940) -> ()  [unwired: 2 in, 2 out]
                                n616 = property on="Sample Channel\nFlow" class="Bool (strict)"("Val(Sgnl)"=FALSE ("Value (Signaling)")) -> ()  [unwired: 2 in, 2 out]
                                }
                                frame True {
                                }
                              }
                            }
                          }
                        }
                        frame #1 {
                          # "For turning on green laser before stage reaches lower spot"
                          n617 = case shown="True" "Green ON\nafter start\nreturn?" {
                            frame False {
                            }
                            frame True {
                              n618 = flat-sequence {
                                frame #0 {
                                n619 = Multiply(x="Green delay after \nstart return (s)", y=1000.0) -> (x*y=w950:dbl)
                                n620 = Wait (ms)(milliseconds to wait=w950) -> ()  [unwired: 1 out]
                                }
                                frame #1 {
                                n621 = property on="Green Laser ON" class="Bool (strict)"("Val(Sgnl)"=TRUE ("Value (Signaling)")) -> ()  [unwired: 2 in, 2 out]
                                }
                              }
                            }
                          }
                          n622 = local read "Saved Stage Positions"() -> (w948:dbl[][])
                          n623 = local write "Cancel dwell"(FALSE ("Cancel dwell")) -> ()
                          n624 = call "move to saved stage position.vi"("error in"=w944, "Stage VISA resource name in"=w945, "Position"="Return Stage \nPosition", "Saved Stage Positions"=w948) -> ("error out"=w946:errorcluster)  [unwired: 1 out]
                          n625 = local write "Stage Control Serial Error"(w946) -> ()
                        }
                        frame #2 {
                          n626 = property on="Trap Pos. FB ON" class="Bool (strict)"("Val(Sgnl)"=w953) -> ()  [unwired: 2 in, 2 out]
                          n627 = case shown="True" "Green ON \nafter return?" {
                            frame False {
                            }
                            frame True {
                              n628 = property on="Green Laser ON" class="Bool (strict)"("Val(Sgnl)"=TRUE ("Value (Signaling)")) -> ()  [unwired: 2 in, 2 out]
                            }
                          }
                          n629 = case shown="True" "Move trap after return?" {
                            frame False {
                            }
                            frame True {
                              n630 = property on="Trap Delta (MHz)" class="DigNum (strict)"("Val(Sgnl)"="Dip Trap Delta 2 (MHz)") -> ()  [unwired: 2 in, 2 out]
                            }
                          }
                          n631 = case shown="True" "Save data after return?" {
                            frame False {
                            }
                            frame True {
                              n632 = property on="Start Saving" class="Bool (strict)"("Val(Sgnl)"=TRUE ("Value (Signaling)")) -> ()  [unwired: 2 in, 2 out]
                            }
                          }
                          n633 = property on="Sample Channel\nFlow" class="Bool (strict)"("Val(Sgnl)"="Flow ON\nduring daq?") -> ()  [unwired: 2 in, 2 out]
                        }
                        frame #3 {
                          n634 = node-c288() -> (w962:T28)  [unwired: 4 in]
                          n635 = timed-loop {
                            timing: w962 -> [_]
                            timing-out: [_] -> w961
                            i -> [w963]
                            stop <- w965 stop-if-true
                            n636 = node-c288() -> ()  [unwired: 1 in, 1 out]
                            n637 = local read "Dump Beads"() -> (w964:bool)
